vi "getNewValueFromXml.vi"(8 "error in (no error)":errorcluster, 10 "Xml":refnum<class "xmlNode.lvclass">, 11 "ScriptEvent in":refnum<class "ScriptEvent.lvclass">) -> (0 "error out":errorcluster, 2 "Xml out":refnum<class "xmlNode.lvclass">, 3 "ScriptEvent out":refnum<class "ScriptEvent.lvclass">)   [LabVIEW 2011, in "Tools.lvlib" / "Scripting.lvlib" / "ScriptEvent.lvclass"]
uses:
  ScriptEvent.lvclass
  xmlNode/xmlNode.lvclass
  ScriptEvent.lvclass/ScriptEvent.ctl
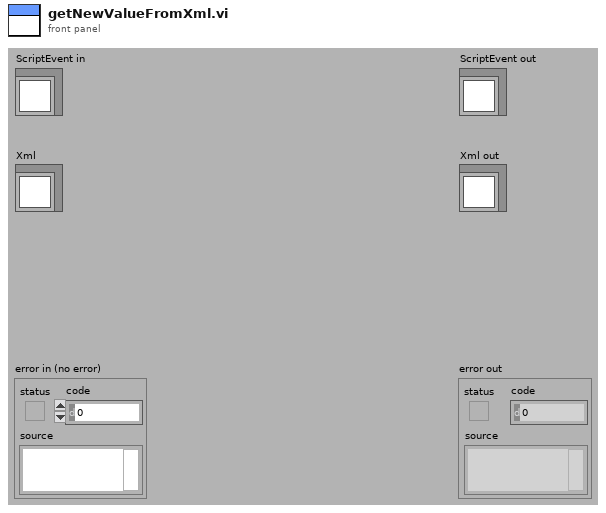
[diagram p1: front panel]
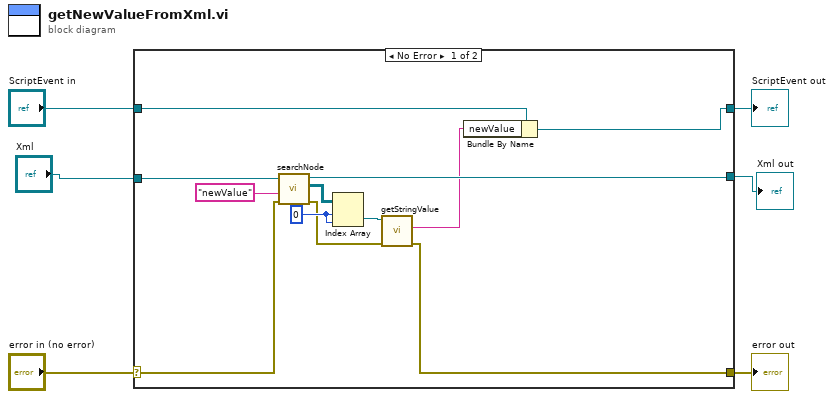
[diagram p0: block diagram]
diagram:
  n1 = case shown="No Error" "error in (no error)" {
    selector: "error in (no error)" -> [w11 w20]
    tunnel: [w7 w20] -> w5
    tunnel: [w9 w19] -> w3
    tunnel: "ScriptEvent in" -> [w10 w19]
    tunnel: "Xml" -> [w13 _]
    tunnel: [w12 _] -> w1
    frame No Error {
      w16 = 0
      n2 = call-dynamic "searchNode.vi"("error in (no error)"=w11, "searchElementName"="newValue", "xmlNode in"=w13) -> ("error out"=w14:errorcluster, "arrayXmlNodes"=w17:refnum<class "xmlNode.lvclass">[][], "xmlNode out"=w12:refnum<class "xmlNode.lvclass">)  [unwired: 6 in]
      n3 = Index Array(array=w17, index (row)=w16, index (col)=w16) -> (element=w15:refnum<class "xmlNode.lvclass">)
      n4 = call-dynamic "getStringValue.vi"("error in (no error)"=w14, "xmlNode.lvclass in"=w15) -> ("error out"=w7:errorcluster, "stringValue"=w8:string)  [unwired: 7 in, 1 out]
      n5 = Bundle By Name(cluster=w10, "newValue"=w8) -> (w9:refnum<class "ScriptEvent.lvclass">)
    }
    frame Error {
    }
  }
  "error out" <- w5
  "ScriptEvent out" <- w3
  "Xml out" <- w1
